vi "EuniceF_LAB6Labview.vi"() -> ()   [LabVIEW 2025]
panel:
  out "Temperature Chart":dbl(graph)
  out "AtoD":i16
  in  "?":bool
  out "Thermomether":dbl(slide) scale=-50.0..50.0 scale format="%1.1f"
  out "Vin":dbl(slide) scale=-10.0..10.0 scale format="%1.1g"
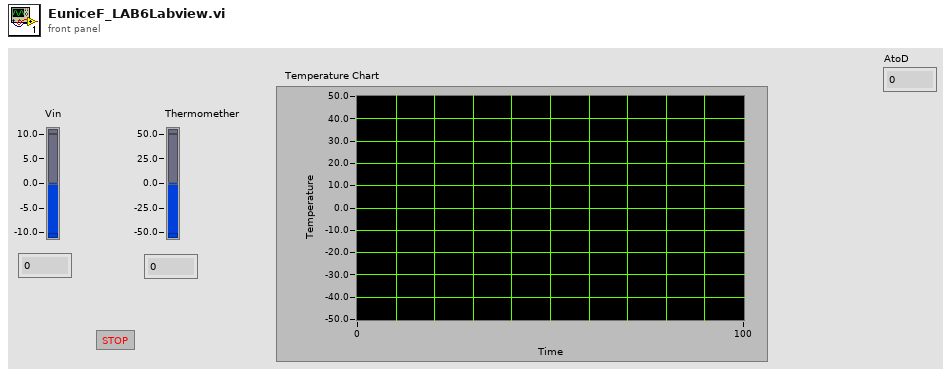
[diagram p1: front panel]
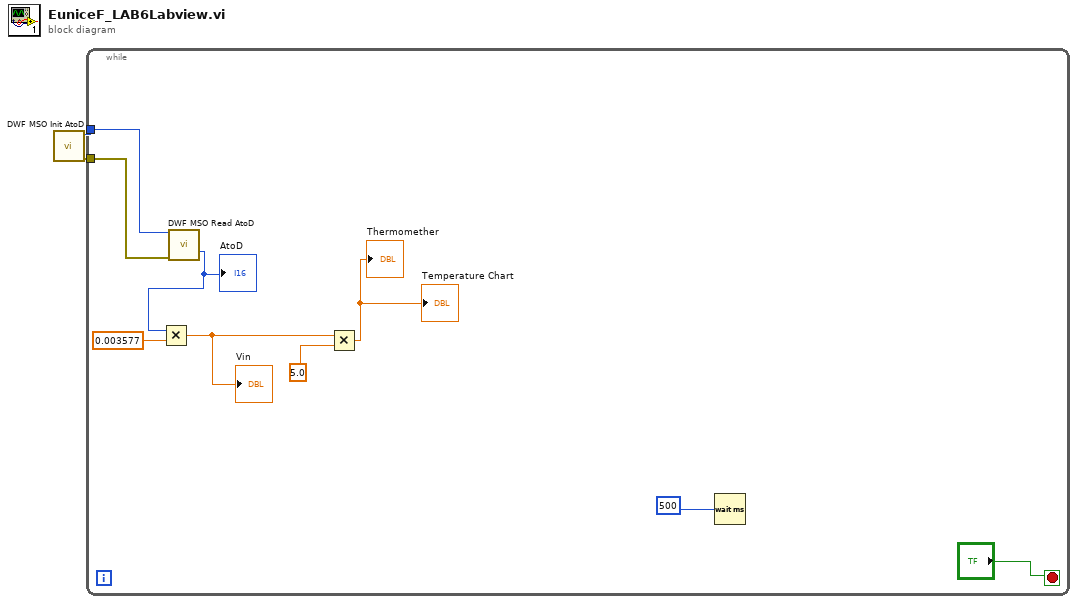
[diagram p0: block diagram]
diagram:
  n1 = call "DWF MSO Init AtoD.vi"() -> ("Error Out"=w1:errorcluster, "Instrument Handle Out"=w2:i32)  [unwired: 10 in]
  n2 = while {
    tunnel: w2 -> [w10]
    tunnel: w1 -> [w9]
    stop <- "?" stop-if-true
    n3 = call "DWF MSO Read AtoD.vi"("Instrument Handle In AtoD"=w10, "Error In"=w9) -> ("AtoD"=w7:i16)  [unwired: 12 in, 1 out]
    "AtoD" <- w7
    n4 = Multiply(x=w7, y=0.003577) -> (x*y=w4:dbl)
    "Vin" <- w4
    n5 = Multiply(x=w4, y=5.0) -> (x*y=→"Thermomether" →"Temperature Chart":dbl)
    n6 = Wait (ms)(milliseconds to wait=u32 500) -> ()  [unwired: 1 out]
  }
